vi "Main Page.vi"(8 "error in (no error)":errorcluster, 11 "Node Ptr":T1 format="%.0x") -> (0 "error out":errorcluster)   [LabVIEW 2017, in "NI-XNET Monitor System Explorer.lvlib"]
uses:
  NI-XNET Monitor System Explorer.lvlib
  <vilib>/NI Veristand/Custom Device API/Custom Device Item Ref.ctl
  <vilib>/NI Veristand/Custom Device API/Custom Device API.lvlib
panel:
  out "Version":string
  in  "SHDocVw.IWebBrowser":refnum<k7>(container)
  in  "Specific Header":cluster{"Section Name":string}={"Section Name"="Custom Device Item Settings"}
  in  "General Header":cluster{"Section Name":string}={"Section Name"="General Custom Device Settings"}
  in  "Description":string
  out "Name":string
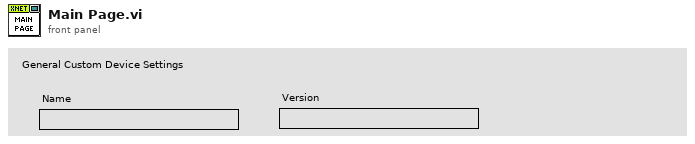
[diagram p1: front panel]
types:
  T1 = typedef "Custom Device API.lvlib/Custom Device Item Ref.ctl" = u64
  T2 = typedef "Custom Device API.lvlib/Custom Device Item Info.ctl" = cluster{"Name":string, "Is Channel":bool, "GUID":string, "Is Waveform":bool}
  T3 = typedef "Custom Device API.lvlib/Custom Device Commands.ctl" = enum16{"Default", "Item renamed", "Shutdown", "Dynamic button pressed"}
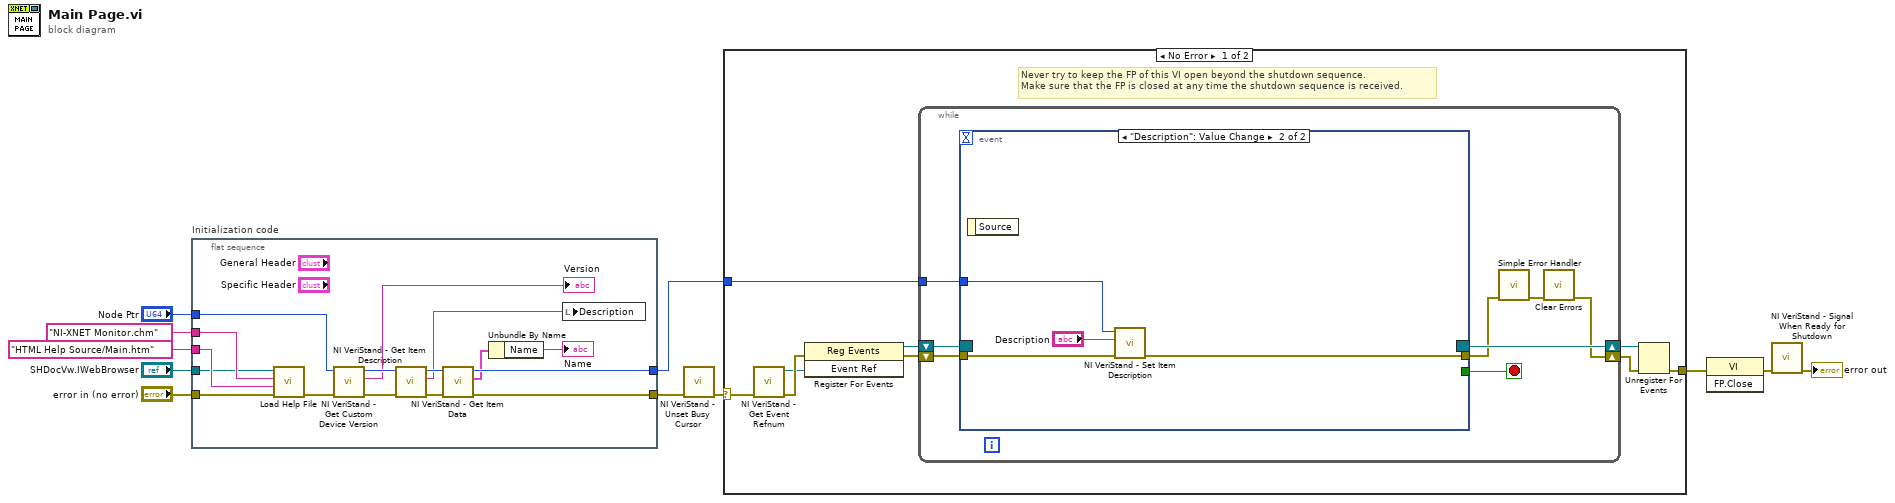
[diagram p0: block diagram]
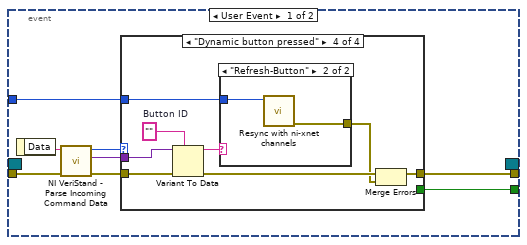
[diagram p2: hidden frame]
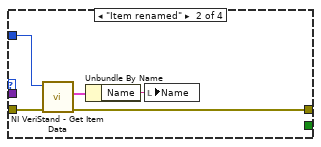
[diagram p4: hidden frame]
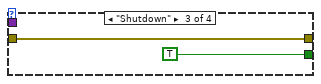
[diagram p5: hidden frame]
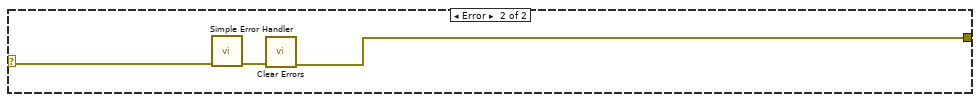
[diagram p7: hidden frame]
diagram:
  n1 = flat-sequence "Initialization code" {
    tunnel: "error in (no error)" -> [w17]
    tunnel: "Node Ptr" -> [w22]
    tunnel: [w23] -> w7
    tunnel: [w27] -> w4
    tunnel: "SHDocVw.IWebBrowser" -> [w14]
    tunnel: "HTML Help Source/Main.htm" ("HTML File") -> [w16]
    tunnel: "NI-XNET Monitor.chm" ("CD_CHM_FileName") -> [w15]
    frame #0 {
      n2 = call "Load Help File.vi"("error in (no error)"=w17, "HTML File to Load"=w16, "Main CHM File"=w15, "Browser"=w14) -> ("error out"=w18:errorcluster)  [unwired: 7 in]
      n3 = call <vilib>:"NI VeriStand - Get Custom Device Version.vi"("error in (no error)"=w18, "Device Ref in"=w22) -> ("error out"=w21:errorcluster, "Value"=→"Version":string, "Device Ref out"=w20:T1)  [unwired: 7 in]
      n4 = call <vilib>:"NI VeriStand - Get Item Description.vi"("error in (no error)"=w21, "Item Ref in"=w20) -> ("error out"=w25:errorcluster, "Description"=w13:string, "Item Ref out"=w26:T1)  [unwired: 7 out]
      n5 = call <vilib>:"NI VeriStand - Get Item Data.vi"("error in (no error)"=w25, "Item Ref in"=w26) -> ("error out"=w23:errorcluster, "Item Info"=w24:T2, "Item Ref out"=w27:T1)  [unwired: 7 out]
      n6 = Unbundle By Name(w24) -> ("Name"=→"Name":string)
      n7 = local write "Description"(w13) -> ()
    }
  }
  n8 = call <vilib>:"NI VeriStand - Unset Busy Cursor.vi"("error in (no error)"=w7) -> ("error out"=w6:errorcluster)  [unwired: 10 out]
  n9 = case shown="No Error" w6 {
    selector: w6 -> [w28 w77]
    tunnel: [w33 w75] -> w11
    tunnel: w4 -> [w29 _]
    frame No Error {
      # "Never try to keep the FP of this VI open beyond the shutdown sequence.\nMake sure that the FP is closed at any time the shutdown sequence is received."
      n10 = call <vilib>:"NI VeriStand - Get Event Refnum.vi"("error in (no error)"=w28) -> ("error out"=w36:errorcluster, "Event Ref"=w32:refnum<user-event>)  [unwired: 9 out]
      n11 = register-events(error in=w36, w32) -> (reference out=w30:refnum<event-registration>, error out=w31:errorcluster)  [unwired: 1 in]
      n12 = while {
        tunnel: w29 -> [w40]
        shift-right: [w37] -> w34
        shift-left: w31 -> [w43]
        shift-right: [w44] -> w35
        shift-left: w30 -> [w42]
        stop <- w41 stop-if-true
        n13 = event shown="[1] \"Description\": Value Change" {
          selector: w42 -> [_ _]
          dyn-events: [_ _] -> w44
          timeout: _ -> [_ _]
          tunnel: w43 -> [w52 w73]
          tunnel: [w48 _] -> w41
          tunnel: [w47 w72] -> w39
          tunnel: w40 -> [w46 w74]
          event User Event {
            n14 = event-data() -> ("Data"=w51:string)  [unwired: 1 out]
            n15 = call <vilib>:"NI VeriStand - Parse Incoming Command Data.vi"("error in (no error)"=w52, "Incoming data"=w51) -> ("error out"=w50:errorcluster, "Outgoing data"=w45:variant, "Action"=w49:T3)  [unwired: 7 out]
            n16 = case shown="\"Dynamic button pressed\"" w49 {
              tunnel: w50 -> [w53 w58 w59 w68]
              tunnel: [_ _ TRUE _] -> w48
              tunnel: [w53 w55 w59 w62] -> w47
              tunnel: w46 -> [_ w57 _ w63]
              tunnel: w45 -> [_ _ _ w67]
              frame "Default", Default {
              }
              frame "Item renamed" {
                n17 = call <vilib>:"NI VeriStand - Get Item Data.vi"("error in (no error)"=w58, "Item Ref in"=w57) -> ("error out"=w55:errorcluster, "Item Info"=w56:T2)  [unwired: 8 out]
                n18 = Unbundle By Name(w56) -> ("Name"=w54:string)
                n19 = local write "Name"(w54) -> ()
              }
              frame "Shutdown" {
              }
              frame "Dynamic button pressed" {
                w66 = ""  # Button ID
                n20 = Variant To Data(error in=w68, type=w66, Variant=w67) -> (data=w64:string, error out=w65:errorcluster)
                n21 = case shown="\"Refresh-Button\"" w64 {
                  tunnel: w63 -> [_ w70]
                  tunnel: [_ w69] -> w61
                  frame Default {
                  }
                  frame "Refresh-Button" {
                    n22 = call "Resync with ni-xnet channels.vi"("Device Item Ref in in"=w70) -> ("Error Out"=w69:errorcluster)  [unwired: 9 in, 1 out]
                  }
                }
                n23 = Merge Errors(w65, w61) -> (w62:errorcluster)
              }
            }
          }
          event "Description": Value Change {
            n24 = event-data() -> ()  [unwired: 2 out]
            n25 = call <vilib>:"NI VeriStand - Set Item Description.vi"("error in (no error)"=w73, "Description"="Description", "Item Ref in"=w74) -> ("error out"=w72:errorcluster)  [unwired: 8 out]
          }
        }
        n26 = call <vilib>:"Simple Error Handler.vi"("error in (no error)"=w39) -> ("error out"=w38:errorcluster)  [unwired: 1 in, 7 out]
        n27 = call <vilib>:"Clear Errors.vi"("error in (no error)"=w38) -> ("error out"=w37:errorcluster)  [unwired: 1 in, 5 out]
      }
      n28 = Unregister For Events(event registration refnum=w35, error in=w34) -> (error out=w33:errorcluster)
    }
    frame Error {
      n29 = call <vilib>:"Simple Error Handler.vi"("error in (no error)"=w77) -> ("error out"=w76:errorcluster)  [unwired: 1 in, 7 out]
      n30 = call <vilib>:"Clear Errors.vi"("error in (no error)"=w76) -> ("error out"=w75:errorcluster)  [unwired: 1 in, 5 out]
    }
  }
  n31 = invoke class="VI" method="FP.Close"(error in=w11) -> (error out=w10:errorcluster)  [unwired: 2 in, 2 out]
  n32 = call <vilib>:"NI VeriStand - Signal When Ready for Shutdown.vi"("error in (no error)"=w10) -> ("error out"=→"error out":errorcluster)  [unwired: 10 out]
